vi "test Group Hardware Channel Info by Transfer Type.vi"(8 "error in":errorcluster, 11 "TestCase in":refnum<class "Engine.lvclass">) -> (0 "error out":errorcluster, 3 "TestCase out":refnum<class "Engine.lvclass">)   [LabVIEW 2020, in "Engine.lvclass"]
uses:
  Engine.lvclass
  <vilib>/addons/_JKI Toolkits/VI Tester/TestCase.llb/TestCase.lvclass
  <vilib>/NI VeriStand/Custom Device API/Custom Device Item Ref.ctl
  <vilib>/NI VeriStand/Custom Device API/Custom Device API.lvlib
  <vilib>/NI VeriStand/Custom Device API/Data Reference.ctl
  Shared/Transfer Type.ctl
  <vilib>/NI VeriStand/Custom Device API/Block Data Reference.ctl
  Encoding and Decoding/Encoding.ctl
  Encoding and Decoding/Encoding and Decoding.lvlib
  Shared/Parameter Definition.ctl
  Shared/RT Parameters.ctl
  Shared/Label.ctl
  Shared/RT Label Settings.ctl
  Shared/RT Hardware Channel Settings.ctl
  System Explorer/Implementation/Implementation.lvlib
  C:/Program Files (x86)/National Instruments/LabVIEW 2020/vi.lib/addons/_JKI Toolkits/VI Tester/TestCase.llb/TestCase.lvclass
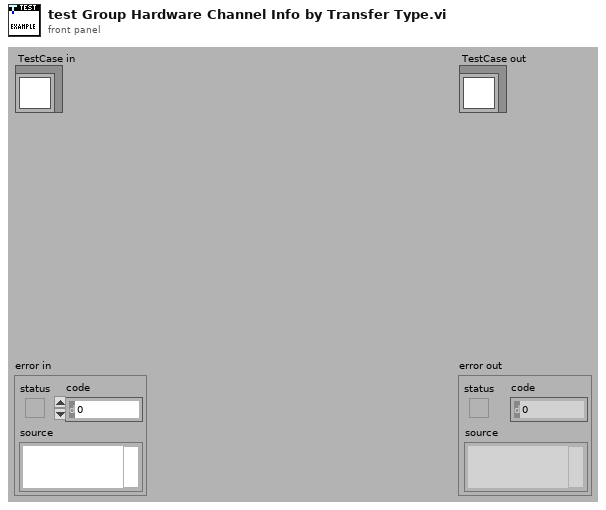
[diagram p1: front panel]
types:
  T1 = typedef "Custom Device API.lvlib/Custom Device Item Ref.ctl" = u64
  T2 = typedef "RT Hardware Channel Settings.ctl" = cluster{"channel #":u16, "channel handle":u64, "labels settings for RT":T3[]}
  T3 = typedef "RT Label Settings.ctl" = cluster{"Name":string, "xmlName":string, "label":T4, "transfer period":u32, "SDI_Enabled":bool, "SDI":u8, "parameter driver data":T5, "transfer type":T10, "has timestamp?":bool, "Label Disable/Trigger Channel Reference":T1, "Message Handle":u64, "Initialized?":bool, "Word Initial Raw Value":u32, "Label Timestamp Channel Data Reference":T9}
  T4 = typedef "Label.ctl" = u8
  T5 = typedef "RT Parameters.ctl" = cluster{"parameter definitions":T6[], "Rx block data refs":T8[], "Rx values":dbl[], "Tx parameter refs":T1[]}
  T6 = typedef "Parameter Definition.ctl" = cluster{"start index":i32, "size":i32, "encoding":T7, "signed":bool, "scale multiplier":dbl, "scale offset":dbl}
  T7 = typedef "Encoding and Decoding.lvlib/Encoding.ctl" = enum16{"BNR", "BCD", "Discrete"}
  T8 = typedef "Custom Device API.lvlib/Block Data Reference.ctl" = cluster{"Data Reference":T9, "Offset":u64, "Length":u64}
  T9 = typedef "Custom Device API.lvlib/Data Reference.ctl" = i32
  T10 = typedef "Transfer Type.ctl" = enum16{"Scheduled", "Acyclic", "Block", "Strobe"}
  T11 = cluster{"Name":string, "Type":enum16{"Output/Write", "Input/Read", "Input/ReadWrite"}, "VS Refs":T1[], "hardware channel data":T2[]}[]
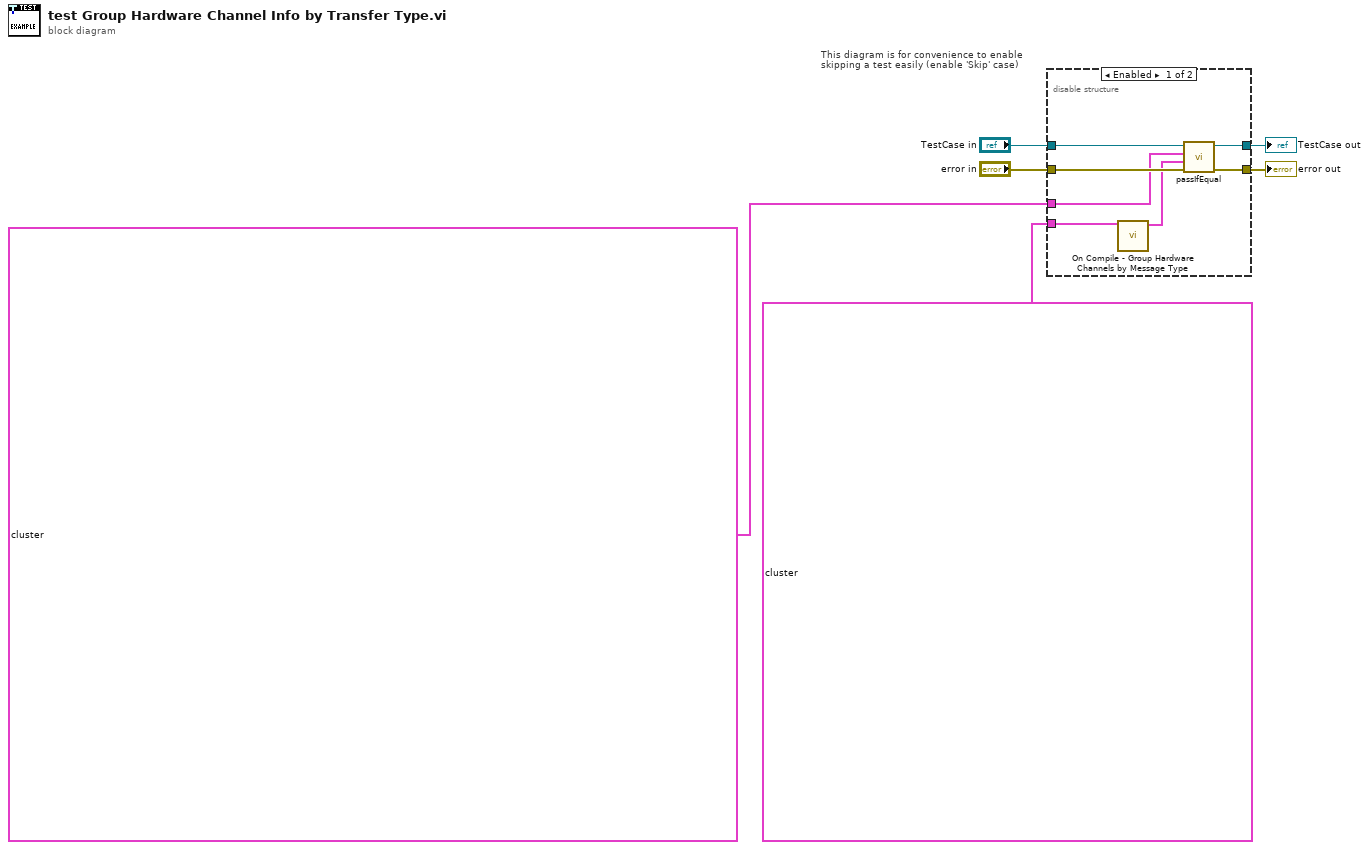
[diagram p0: block diagram]
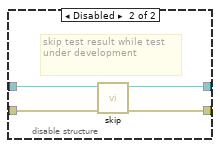
[diagram p2: hidden frame]
diagram:
  n1 = disable-structure "This diagram is for convenience to enable skipping a test easily (enable 'Skip' case)" shown="Enabled" {
    disable-tunnel: "TestCase in" -> [w13 w17]
    disable-tunnel: [w10 w15] -> w3
    disable-tunnel: [w9 w16] -> w5
    disable-tunnel: "error in" -> [w12 w14]
    disable-tunnel: T2[] [{"channel #"=17, "channel handle"=0, "labels settings for RT"=[{"Name"="label 134", "xmlName"="134", "label"=134, "transfer period"=0, "SDI_Enabled"=FALSE, "SDI"=0, "parameter driver data"={"parameter definitions"=[{"start index"=18, "size"=10, "encoding"=enum."BNR", "signed"=TRUE, "scale multiplier"=16.0, "scale offset"=0.0}], "Rx block data refs"=[], "Rx values"=[], "Tx parameter refs"=[171340]}, "transfer type"=enum."Scheduled", "has timestamp?"=FALSE, "Label Disable/Trigger Channel Reference"=18446744073709551615, "Message Handle"=0, "Initialized?"=FALSE, "Word Initial Raw Value"=0, "Label Timestamp Channel Data Reference"=0}]}, {"channel #"=19, "channel handle"=0, "labels settings for RT"=[{"Name"="label 135", "xmlName"="135", "label"=135, "transfer period"=0, "SDI_Enabled"=FALSE, "SDI"=0, "parameter driver data"={"parameter definitions"=[{"start index"=10, "size"=19, "encoding"=enum."BCD", "signed"=TRUE, "scale multiplier"=1.0, "scale offset"=0.0}], "Rx block data refs"=[], "Rx values"=[], "Tx parameter refs"=[191350]}, "transfer type"=enum."Acyclic", "has timestamp?"=FALSE, "Label Disable/Trigger Channel Reference"=18446744073709551615, "Message Handle"=0, "Initialized?"=FALSE, "Word Initial Raw Value"=0, "Label Timestamp Channel Data Reference"=0}]}, {"channel #"=21, "channel handle"=0, "labels settings for RT"=[{"Name"="label 136", "xmlName"="136", "label"=136, "transfer period"=0, "SDI_Enabled"=FALSE, "SDI"=0, "parameter driver data"={"parameter definitions"=[{"start index"=13, "size"=16, "encoding"=enum."BNR", "signed"=TRUE, "scale multiplier"=1.0, "scale offset"=0.0}, {"start index"=10, "size"=1, "encoding"=enum."Discrete", "signed"=FALSE, "scale multiplier"=1.0, "scale offset"=0.0}, {"start index"=11, "size"=1, "encoding"=enum."Discrete", "signed"=FALSE, "scale multiplier"=1.0, "scale offset"=0.0}], "Rx block data refs"=[], "Rx values"=[], "Tx parameter refs"=[211360, 211361, 211362]}, "transfer type"=enum."Scheduled", "has timestamp?"=FALSE, "Label Disable/Trigger Channel Reference"=18446744073709551615, "Message Handle"=0, "Initialized?"=FALSE, "Word Initial Raw Value"=0, "Label Timestamp Channel Data Reference"=0}]}] ("Rx hardware channel data") -> [w8 _]
    disable-tunnel: T11 [{"Name"="Asynchronous - Tx Channels - Cyclic Labels - Disable/Enable Channels", "Type"=enum."Input/Read", "VS Refs"=[18446744073709551615, 18446744073709551615], "hardware channel data"=[{"channel #"=17, "channel handle"=0, "labels settings for RT"=[{"Name"="label 134", "xmlName"="134", "label"=134, "transfer period"=0, "SDI_Enabled"=FALSE, "SDI"=0, "parameter driver data"={"parameter definitions"=[], "Rx block data refs"=[], "Rx values"=[], "Tx parameter refs"=[171340]}, "transfer type"=enum."Scheduled", "has timestamp?"=FALSE, "Label Disable/Trigger Channel Reference"=18446744073709551615, "Message Handle"=0, "Initialized?"=FALSE, "Word Initial Raw Value"=0, "Label Timestamp Channel Data Reference"=0}]}, {"channel #"=21, "channel handle"=0, "labels settings for RT"=[{"Name"="label 136", "xmlName"="136", "label"=136, "transfer period"=0, "SDI_Enabled"=FALSE, "SDI"=0, "parameter driver data"={"parameter definitions"=[], "Rx block data refs"=[], "Rx values"=[], "Tx parameter refs"=[211360, 211361, 211362]}, "transfer type"=enum."Scheduled", "has timestamp?"=FALSE, "Label Disable/Trigger Channel Reference"=18446744073709551615, "Message Handle"=0, "Initialized?"=FALSE, "Word Initial Raw Value"=0, "Label Timestamp Channel Data Reference"=0}]}]}, {"Name"="Asynchronous - Tx Channels - Acyclic Labels - Trigger Channels", "Type"=enum."Input/ReadWrite", "VS Refs"=[18446744073709551615], "hardware channel data"=[{"channel #"=19, "channel handle"=0, "labels settings for RT"=[{"Name"="label 135", "xmlName"="135", "label"=135, "transfer period"=0, "SDI_Enabled"=FALSE, "SDI"=0, "parameter driver data"={"parameter definitions"=[], "Rx block data refs"=[], "Rx values"=[], "Tx parameter refs"=[191350]}, "transfer type"=enum."Acyclic", "has timestamp?"=FALSE, "Label Disable/Trigger Channel Reference"=18446744073709551615, "Message Handle"=0, "Initialized?"=FALSE, "Word Initial Raw Value"=0, "Label Timestamp Channel Data Reference"=0}]}]}, {"Name"="Asynchronous - Tx Channels - Scheduled Labels - Parameters", "Type"=enum."Input/Read", "VS Refs"=[171340, 211360, 211361, 211362], "hardware channel data"=[{"channel #"=17, "channel handle"=0, "labels settings for RT"=[{"Name"="label 134", "xmlName"="134", "label"=134, "transfer period"=0, "SDI_Enabled"=FALSE, "SDI"=0, "parameter driver data"={"parameter definitions"=[{"start index"=18, "size"=10, "encoding"=enum."BNR", "signed"=TRUE, "scale multiplier"=16.0, "scale offset"=0.0}], "Rx block data refs"=[], "Rx values"=[], "Tx parameter refs"=[171340]}, "transfer type"=enum."Scheduled", "has timestamp?"=FALSE, "Label Disable/Trigger Channel Reference"=18446744073709551615, "Message Handle"=0, "Initialized?"=FALSE, "Word Initial Raw Value"=0, "Label Timestamp Channel Data Reference"=0}]}, {"channel #"=21, "channel handle"=0, "labels settings for RT"=[{"Name"="label 136", "xmlName"="136", "label"=136, "transfer period"=0, "SDI_Enabled"=FALSE, "SDI"=0, "parameter driver data"={"parameter definitions"=[{"start index"=13, "size"=16, "encoding"=enum."BNR", "signed"=TRUE, "scale multiplier"=1.0, "scale offset"=0.0}, {"start index"=10, "size"=1, "encoding"=enum."Discrete", "signed"=FALSE, "scale multiplier"=1.0, "scale offset"=0.0}, {"start index"=11, "size"=1, "encoding"=enum."Discrete", "signed"=FALSE, "scale multiplier"=1.0, "scale offset"=0.0}], "Rx block data refs"=[], "Rx values"=[], "Tx parameter refs"=[211360, 211361, 211362]}, "transfer type"=enum."Scheduled", "has timestamp?"=FALSE, "Label Disable/Trigger Channel Reference"=18446744073709551615, "Message Handle"=0, "Initialized?"=FALSE, "Word Initial Raw Value"=0, "Label Timestamp Channel Data Reference"=0}]}]}, {"Name"="Asynchronous - Tx Channels - Acyclic Labels - Parameters", "Type"=enum."Input/Read", "VS Refs"=[191350], "hardware channel data"=[{"channel #"=19, "channel handle"=0, "labels settings for RT"=[{"Name"="label 135", "xmlName"="135", "label"=135, "transfer period"=0, "SDI_Enabled"=FALSE, "SDI"=0, "parameter driver data"={"parameter definitions"=[{"start index"=10, "size"=19, "encoding"=enum."BCD", "signed"=TRUE, "scale multiplier"=1.0, "scale offset"=0.0}], "Rx block data refs"=[], "Rx values"=[], "Tx parameter refs"=[191350]}, "transfer type"=enum."Acyclic", "has timestamp?"=FALSE, "Label Disable/Trigger Channel Reference"=18446744073709551615, "Message Handle"=0, "Initialized?"=FALSE, "Word Initial Raw Value"=0, "Label Timestamp Channel Data Reference"=0}]}]}] ("grouped hardware channel data refs") -> [w7 _]
    frame Enabled {
      n2 = call "On Compile - Group Hardware Channels by Message Type.vi"("hardware channel data"=w8) -> ("grouped hardware channel data refs"=w11:T11)  [unwired: 9 in, 1 out]
      n3 = call-dynamic "passIfEqual.vi"("error in (no error)"=w12, "y"=w11, "x"=w7, "TestCase in"=w13) -> ("error out"=w9:errorcluster, "TestCase out"=w10:refnum<class "Engine.lvclass">)  [unwired: 6 in]
    }
    frame Disabled {
      # "skip test result while test under development"
      n4 = call <vilib>:"skip.vi"("error in (no error)"=w14, "TestCase in"=w17) -> ("error out"=w16:errorcluster, "TestCase out"=w15:refnum<class "Engine.lvclass">)  [unwired: 8 in]
    }
  }
  "error out" <- w5
  "TestCase out" <- w3
